vi "PH_Tektronix_7000.Configure Channel.vi"(0 "i ref in":refnum<vi>, 1 "Channel":u16(ring) items=["Channel 1", "Channel 2", "Channel 3", "Channel 4", "Math 1", "Math 2", "Math 3", "Math 4", "Reference 1", "Reference 2", "Reference 3", "Reference 4"], 2 "Channel Configuration":T1={"Enable Channel"=FALSE, "Bandwidth"=0, "Input Impedance"=0, "Vertical Coupling"=0, "Probe Attenuation"=1.0, "Range [V/div]"=1.0, "Position [div]"=10.0, "Bandwidth raw"=""} {"Vertical Coupling" items=["AC", "DC", "Ground"]; "Input Impedance" items=["1M", "50"]; "Bandwidth" items=["FULL", "500 MHz", "250 MHz", "150 MHz", "20 MHz"]}, 5 "error IO":errorcluster) -> (14 "i ref out":refnum<vi>, 19 "error out":errorcluster)   [LabVIEW 2014, in "PH_Tektronix_7000.lvlib"]
doc: "If the connection is established, the channel configuration is set and written to own attributes as well as the errors."
uses:
  PH_Tektronix_7000.lvlib
  PH_Tektronix_7000.Channel Config.ctl
  instr.lib/Tektronix7000Series/Tektronix 7000 Series - Driver np.lvlib
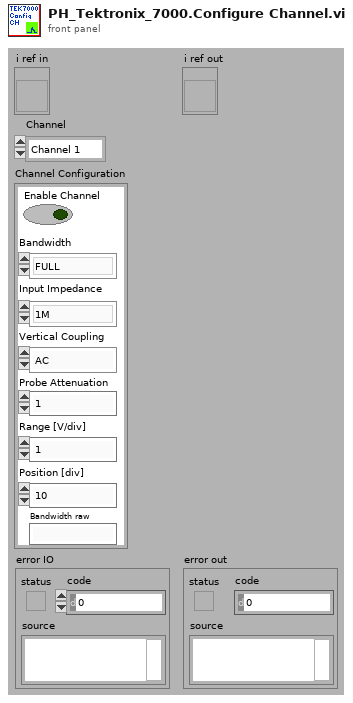
[diagram p1: front panel]
types:
  T1 = typedef "PH_Tektronix_7000.lvlib/PH_Tektronix_7000.Channel Config.ctl" = cluster{"Enable Channel":bool, "Bandwidth":u16, "Input Impedance":u16, "Vertical Coupling":u16, "Probe Attenuation":dbl, "Range [V/div]":dbl, "Position [div]":dbl, "Bandwidth raw":string}
  T2 = typedef "PH_Tektronix_7000.lvlib/PH_Tektronix_7000.i attribute.ctl" = cluster{"VISA Resource Name":refnum<visa-resource-name>, "IDN":cluster{"Instrument Driver":string, "Instrument Firmware":string, "Model":string, "Serial Number":string}, "Selftest":cluster{"Result":i32, "Message":string}, "Trigger Configuration":T3, "Acquisition Configuration":T4, "GUI Refs":T5, "State":T6, "Error Message":string, "Allow Prdc Loop?":bool, "Channel 1":T1, "Channel 2":T1, "Channel 3":T1, "Channel 4":T1, "Data CH 1":waveform(dbl), "Data CH 2":waveform(dbl), "Data CH 3":waveform(dbl), "Data CH 4":waveform(dbl), "Allow config?":bool, "Name Channel 1":string, "Name Channel 2":string, "Name Channel 3":string, "Name Channel 4":string, "Fetch Data before sending to PSDB?":bool, "Constructor passed?":bool, "Data taken at":timestamp, "Plot Colors":u32[], "Default VISA Resource":string}
  T3 = typedef "PH_Tektronix_7000.lvlib/PH_Tektronix_7000.Trigger Config.ctl" = cluster{"Source":u16, "Level [V]":dbl, "Slope":u16, "Coupling":u16, "Trigger Mode":u16}
  T4 = typedef "PH_Tektronix_7000.lvlib/PH_Tektronix_7000.Acquisition Config.ctl" = cluster{"Record Length":u32, "Timebase [s/div]":dbl, "Position [%]":dbl, "Acquisition Type":u16, "Average Waveforms":i32, "Envelope Waveforms":i32, "WfmDB Samples":i32, "Continuous?":bool, "Delay [s]":dbl, "Run?":bool}
  T5 = typedef "PH_Tektronix_7000.lvlib/PH_Tektronix_7000.GUI Refs.ctl" = cluster{"Graph":refnum<vi>, "State":refnum<vi>, "Delete":refnum<vi>, "VISA Resource":refnum<vi>, "Allow Configure":refnum<vi>, "Fetch Data":refnum<vi>, "Fetch before sending Data to PSDB":refnum<vi>, "Name Channel 1":refnum<vi>, "Name Channel 2":refnum<vi>, "Name Channel 3":refnum<vi>, "Name Channel 4":refnum<vi>, "Prdc Intervall [ms]":refnum<vi>, "Data taken":refnum<vi>, "Model":refnum<vi>, "Serial Number":refnum<vi>, "Firmware":refnum<vi>, "Driver":refnum<vi>, "Acquisition":refnum<vi>, "Trigger":refnum<vi>, "Cursor: D Time [s]":refnum<vi>, "Cursor: D Signal [V]":refnum<vi>, "Channel 1":refnum<vi>, "Channel 2":refnum<vi>, "Channel 3":refnum<vi>, "Channel 4":refnum<vi>}
  T6 = typedef "PH_StatusHandler.lvlib/PH_StatusHandler.Status.ctl" = i16
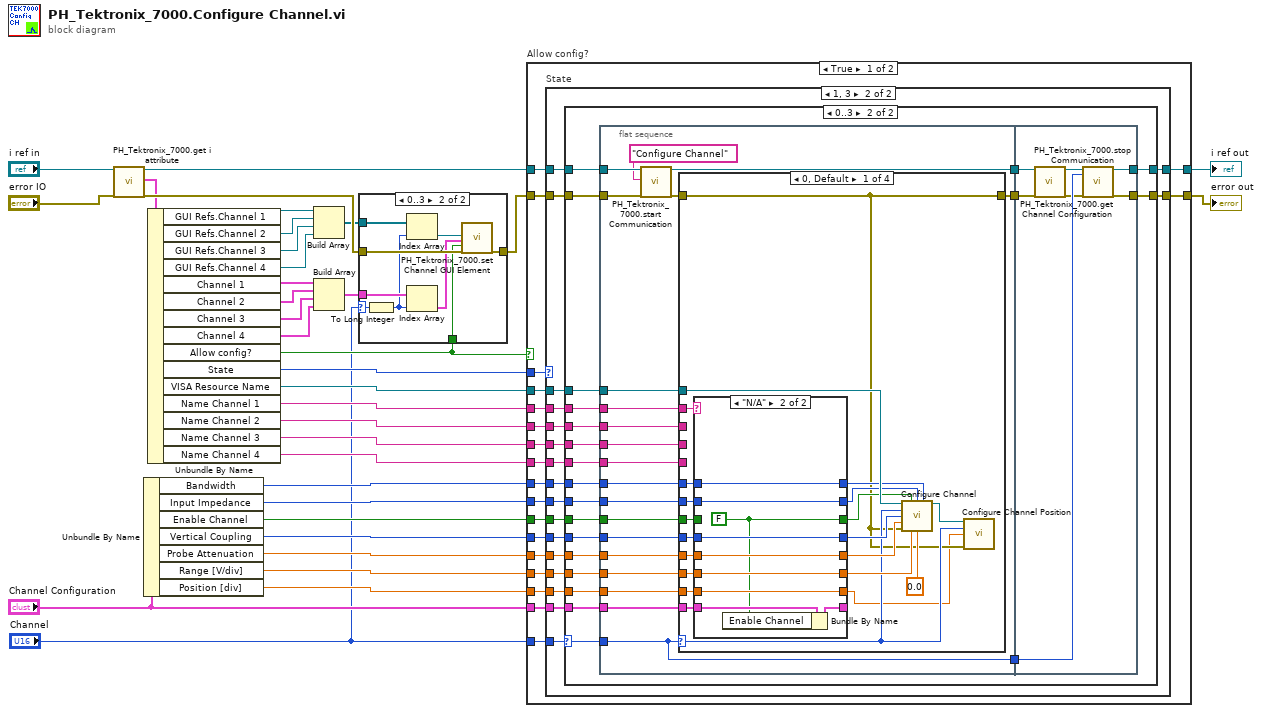
[diagram p0: block diagram]
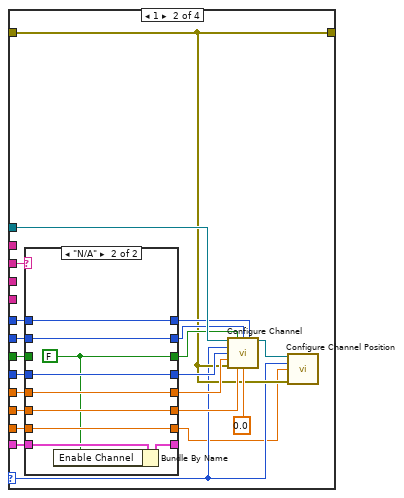
[diagram p6: hidden frame]
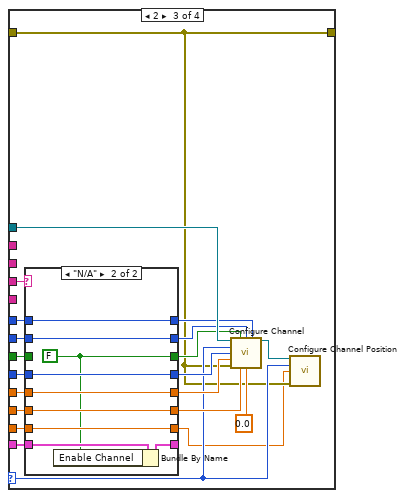
[diagram p8: hidden frame]
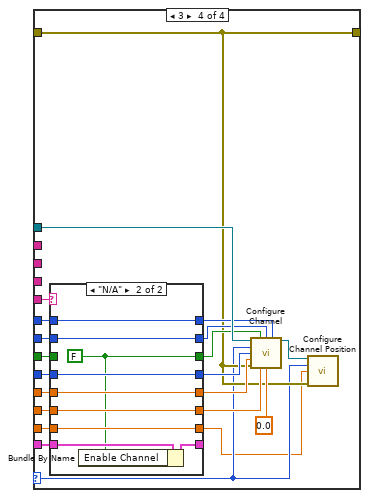
[diagram p10: hidden frame]
diagram:
  n1 = call "PH_Tektronix_7000.get i attribute.vi"("i ref in"="i ref in", "error in (no error)"="error IO") -> ("i ref out"=w30:refnum<vi>, "i attribute"=w32:T2, "error out"=w33:errorcluster)  [unwired: 15 in]
  n2 = Unbundle By Name("Channel Configuration") -> ("Bandwidth"=w27:u16, "Input Impedance"=w26:u16, "Enable Channel"=w25:bool, "Vertical Coupling"=w24:u16, "Probe Attenuation"=w23:dbl, "Range [V/div]"=w22:dbl, "Position [div]"=w21:dbl)
  n3 = Unbundle By Name(w32) -> ("GUI Refs.Channel 1"=w5:refnum<vi>, "GUI Refs.Channel 2"=w3:refnum<vi>, "GUI Refs.Channel 3"=w2:refnum<vi>, "GUI Refs.Channel 4"=w1:refnum<vi>, "Channel 1"=w7:T1, "Channel 2"=w10:T1, "Channel 3"=w9:T1, "Channel 4"=w8:T1, "Allow config?"=w12:bool, "State"=w13:T6, "VISA Resource Name"=w14:refnum<visa-resource-name>, "Name Channel 1"=w19:string, "Name Channel 2"=w18:string, "Name Channel 3"=w17:string, "Name Channel 4"=w16:string)
  n4 = Build Array(w5, w3, w2, w1) -> (w4:refnum<vi>[])
  n5 = Build Array(w7, w10, w9, w8) -> (w6:T1[])
  n6 = case shown="0..3" "Channel" {
    selector: "Channel" -> [_ w38]
    tunnel: w33 -> [w35 w44]
    tunnel: [w35 w43] -> w15
    tunnel: w12 -> [_ w42]
    tunnel: w4 -> [_ w41]
    tunnel: w6 -> [_ w40]
    frame Default {
    }
    frame 0..3 {
      n7 = To Long Integer(number=w38) -> (32bit integer=w36:i32)
      n8 = Index Array(array=w41, index=w36) -> (element=w37:refnum<vi>)
      n9 = Index Array(array=w40, index=w36) -> (element=w39:T1)
      n10 = call "PH_Tektronix_7000.set Channel GUI Element.vi"("GUI Ref Channel"=w37, "Channel Config"=w39, "enabled?"=w42, "error in"=w44) -> ("error out"=w43:errorcluster)  [unwired: 15 in]
    }
  }
  n11 = case "Allow config?" shown="True" w12 {
    tunnel: [w63 w287] -> w34
    tunnel: w15 -> [w62 w286]
    tunnel: w14 -> [w61 _]
    tunnel: w30 -> [w60 w287]
    tunnel: [w59 w286] -> w28
    tunnel: w27 -> [w58 _]
    tunnel: w26 -> [w57 _]
    tunnel: w25 -> [w56 _]
    tunnel: w24 -> [w55 _]
    tunnel: w23 -> [w54 _]
    tunnel: w22 -> [w53 _]
    tunnel: w21 -> [w52 _]
    tunnel: w13 -> [w45 _]
    tunnel: "Channel Configuration" -> [w51 _]
    tunnel: "Channel" -> [w46 _]
    tunnel: w19 -> [w50 _]
    tunnel: w18 -> [w49 _]
    tunnel: w17 -> [w48 _]
    tunnel: w16 -> [w47 _]
    frame True {
      n12 = case "State" shown="1, 3" w45 {
        tunnel: [w65 w66] -> w63
        tunnel: w62 -> [w64 w83]
        tunnel: w61 -> [_ w82]
        tunnel: w60 -> [w65 w67]
        tunnel: [w64 w81] -> w59
        tunnel: w58 -> [_ w80]
        tunnel: w57 -> [_ w79]
        tunnel: w56 -> [_ w78]
        tunnel: w55 -> [_ w77]
        tunnel: w54 -> [_ w76]
        tunnel: w53 -> [_ w75]
        tunnel: w52 -> [_ w74]
        tunnel: w51 -> [_ w73]
        tunnel: w50 -> [_ w72]
        tunnel: w49 -> [_ w71]
        tunnel: w48 -> [_ w70]
        tunnel: w47 -> [_ w69]
        tunnel: w46 -> [_ w68]
        frame Default {
        }
        frame 1, 3 {
          n13 = case shown="0..3" w68 {
            selector: w68 -> [_ w93]
            tunnel: w83 -> [w84 w91]
            tunnel: w82 -> [_ w106]
            tunnel: [w84 w87] -> w81
            tunnel: w80 -> [_ w105]
            tunnel: w79 -> [_ w104]
            tunnel: w78 -> [_ w103]
            tunnel: w77 -> [_ w102]
            tunnel: w76 -> [_ w101]
            tunnel: w75 -> [_ w100]
            tunnel: w74 -> [_ w99]
            tunnel: w73 -> [_ w98]
            tunnel: w72 -> [_ w97]
            tunnel: w71 -> [_ w96]
            tunnel: w70 -> [_ w95]
            tunnel: w69 -> [_ w94]
            tunnel: w67 -> [w85 w92]
            tunnel: [w85 w88] -> w66
            frame Default {
            }
            frame 0..3 {
              n14 = flat-sequence {
                tunnel: w106 -> [w126]
                tunnel: w105 -> [w125]
                tunnel: w104 -> [w124]
                tunnel: w103 -> [w123]
                tunnel: w102 -> [w122]
                tunnel: w101 -> [w121]
                tunnel: w100 -> [w120]
                tunnel: w99 -> [w119]
                tunnel: w98 -> [w118]
                tunnel: w97 -> [w117]
                tunnel: w96 -> [w116]
                tunnel: w95 -> [w115]
                tunnel: w94 -> [w114]
                tunnel: w93 -> [w107]
                tunnel: w92 -> [w113]
                tunnel: w91 -> [w112]
                tunnel: [w109] -> w90
                tunnel: [w108] -> w89
                tunnel: [w107] -> w86
                tunnel: [w284] -> w87
                tunnel: [w283] -> w88
                tunnel: w90 -> [w280]
                tunnel: w89 -> [w285]
                tunnel: w86 -> [w282]
                frame #0 {
                  n15 = call "PH_Tektronix_7000.start Communication.vi"("i ref in"=w113, "Action"="Configure Channel", "error in"=w112) -> ("i ref out"=w109:refnum<vi>, "error out"=w111:errorcluster)  [unwired: 15 in]
                  n16 = case "Channel Label" shown="0, Default" w107 {
                    selector: w107 -> [w130 w166 w205 w242]
                    tunnel: w111 -> [w128 w168 w204 w244]
                    tunnel: w126 -> [w147 w185 w223 w261]
                    tunnel: [w128 w168 w204 w244] -> w108
                    tunnel: w125 -> [w139 w183 w221 w260]
                    tunnel: w124 -> [w140 w182 w220 w259]
                    tunnel: w123 -> [w141 w181 w219 w258]
                    tunnel: w122 -> [w142 w180 w218 w257]
                    tunnel: w121 -> [w143 w179 w217 w256]
                    tunnel: w120 -> [w144 w178 w216 w255]
                    tunnel: w119 -> [w145 w177 w215 w254]
                    tunnel: w118 -> [w146 w176 w214 w253]
                    tunnel: w117 -> [w133 _ _ _]
                    tunnel: w116 -> [_ w184 _ _]
                    tunnel: w115 -> [_ _ w222 _]
                    tunnel: w114 -> [_ _ _ w252]
                    frame 0, Default {
                      n17 = case shown="\"N/A\"" w133 {
                        tunnel: w139 -> [w155 w164]
                        tunnel: [w155 w164] -> w135
                        tunnel: w140 -> [w154 w163]
                        tunnel: [w154 w163] -> w134
                        tunnel: w141 -> [w153 _]
                        tunnel: [w153 w157] -> w136
                        tunnel: w142 -> [w152 w162]
                        tunnel: [w152 w162] -> w132
                        tunnel: w143 -> [w151 w161]
                        tunnel: [w151 w161] -> w137
                        tunnel: w144 -> [w150 w160]
                        tunnel: [w150 w160] -> w138
                        tunnel: w145 -> [w149 w159]
                        tunnel: [w149 w159] -> w127
                        tunnel: w146 -> [w148 w158]
                        tunnel: [w148 w156] -> _
                        frame Default {
                        }
                        frame "N/A" {
                          w157 = FALSE
                          n18 = Bundle By Name(cluster=w158, "Enable Channel"=w157) -> (w156:T1)
                        }
                      }
                      n19 = call "Configure Channel.vi"("VISA resource name"=w147, "Enable Channel (T: Enable)"=w136, "Input Impedance (0: 1M ohm)"=w134, "Bandwidth (0: FULL)"=w135, "Channel (0: Channel 1)"=w130, "Vertical Coupling (1: DC)"=w132, "Probe Attenuation (1.0)"=w137, "error in (no error)"=w128, "Vertical Range (10.0 V)"=w138, "Vertical Offset (0.0 V)"=0.0) -> ("VISA resource name out"=w129:refnum<visa-resource-name>)  [unwired: 4 in, 1 out]
                      n20 = call "Configure Channel Position.vi"("VISA resource name"=w129, "Channel (0: Channel 1)"=w130, "Vertical Position (0.0 div)"=w127, "error in (no error)"=w128) -> ()  [unwired: 10 in, 2 out]
                    }
                    frame 1 {
                      n21 = case shown="\"N/A\"" w184 {
                        tunnel: w183 -> [w193 w202]
                        tunnel: [w193 w202] -> w175
                        tunnel: w182 -> [w192 w201]
                        tunnel: [w192 w201] -> w174
                        tunnel: w181 -> [w191 _]
                        tunnel: [w191 w195] -> w173
                        tunnel: w180 -> [w190 w200]
                        tunnel: [w190 w200] -> w172
                        tunnel: w179 -> [w189 w199]
                        tunnel: [w189 w199] -> w171
                        tunnel: w178 -> [w188 w198]
                        tunnel: [w188 w198] -> w170
                        tunnel: w177 -> [w187 w197]
                        tunnel: [w187 w197] -> w165
                        tunnel: w176 -> [w186 w196]
                        tunnel: [w186 w194] -> _
                        frame Default {
                        }
                        frame "N/A" {
                          w195 = FALSE
                          n22 = Bundle By Name(cluster=w196, "Enable Channel"=w195) -> (w194:T1)
                        }
                      }
                      n23 = call "Configure Channel.vi"("VISA resource name"=w185, "Enable Channel (T: Enable)"=w173, "Input Impedance (0: 1M ohm)"=w174, "Bandwidth (0: FULL)"=w175, "Channel (0: Channel 1)"=w166, "Vertical Coupling (1: DC)"=w172, "Probe Attenuation (1.0)"=w171, "error in (no error)"=w168, "Vertical Range (10.0 V)"=w170, "Vertical Offset (0.0 V)"=0.0) -> ("VISA resource name out"=w167:refnum<visa-resource-name>)  [unwired: 4 in, 1 out]
                      n24 = call "Configure Channel Position.vi"("VISA resource name"=w167, "Channel (0: Channel 1)"=w166, "Vertical Position (0.0 div)"=w165, "error in (no error)"=w168) -> ()  [unwired: 10 in, 2 out]
                    }
                    frame 2 {
                      n25 = case shown="\"N/A\"" w222 {
                        tunnel: w221 -> [w231 w240]
                        tunnel: [w231 w240] -> w213
                        tunnel: w220 -> [w230 w239]
                        tunnel: [w230 w239] -> w212
                        tunnel: w219 -> [w229 _]
                        tunnel: [w229 w233] -> w211
                        tunnel: w218 -> [w228 w238]
                        tunnel: [w228 w238] -> w210
                        tunnel: w217 -> [w227 w237]
                        tunnel: [w227 w237] -> w209
                        tunnel: w216 -> [w226 w236]
                        tunnel: [w226 w236] -> w208
                        tunnel: w215 -> [w225 w235]
                        tunnel: [w225 w235] -> w203
                        tunnel: w214 -> [w224 w234]
                        tunnel: [w224 w232] -> _
                        frame Default {
                        }
                        frame "N/A" {
                          w233 = FALSE
                          n26 = Bundle By Name(cluster=w234, "Enable Channel"=w233) -> (w232:T1)
                        }
                      }
                      n27 = call "Configure Channel.vi"("VISA resource name"=w223, "Enable Channel (T: Enable)"=w211, "Input Impedance (0: 1M ohm)"=w212, "Bandwidth (0: FULL)"=w213, "Channel (0: Channel 1)"=w205, "Vertical Coupling (1: DC)"=w210, "Probe Attenuation (1.0)"=w209, "error in (no error)"=w204, "Vertical Range (10.0 V)"=w208, "Vertical Offset (0.0 V)"=0.0) -> ("VISA resource name out"=w206:refnum<visa-resource-name>)  [unwired: 4 in, 1 out]
                      n28 = call "Configure Channel Position.vi"("VISA resource name"=w206, "Channel (0: Channel 1)"=w205, "Vertical Position (0.0 div)"=w203, "error in (no error)"=w204) -> ()  [unwired: 10 in, 2 out]
                    }
                    frame 3 {
                      n29 = case shown="\"N/A\"" w252 {
                        tunnel: w260 -> [w269 w278]
                        tunnel: [w269 w278] -> w251
                        tunnel: w259 -> [w268 w277]
                        tunnel: [w268 w277] -> w250
                        tunnel: w258 -> [w267 _]
                        tunnel: [w267 w271] -> w249
                        tunnel: w257 -> [w266 w276]
                        tunnel: [w266 w276] -> w248
                        tunnel: w256 -> [w265 w275]
                        tunnel: [w265 w275] -> w247
                        tunnel: w255 -> [w264 w274]
                        tunnel: [w264 w274] -> w246
                        tunnel: w254 -> [w263 w273]
                        tunnel: [w263 w273] -> w241
                        tunnel: w253 -> [w262 w272]
                        tunnel: [w262 w270] -> _
                        frame Default {
                        }
                        frame "N/A" {
                          w271 = FALSE
                          n30 = Bundle By Name(cluster=w272, "Enable Channel"=w271) -> (w270:T1)
                        }
                      }
                      n31 = call "Configure Channel.vi"("VISA resource name"=w261, "Enable Channel (T: Enable)"=w249, "Input Impedance (0: 1M ohm)"=w250, "Bandwidth (0: FULL)"=w251, "Channel (0: Channel 1)"=w242, "Vertical Coupling (1: DC)"=w248, "Probe Attenuation (1.0)"=w247, "error in (no error)"=w244, "Vertical Range (10.0 V)"=w246, "Vertical Offset (0.0 V)"=0.0) -> ("VISA resource name out"=w243:refnum<visa-resource-name>)  [unwired: 4 in, 1 out]
                      n32 = call "Configure Channel Position.vi"("VISA resource name"=w243, "Channel (0: Channel 1)"=w242, "Vertical Position (0.0 div)"=w241, "error in (no error)"=w244) -> ()  [unwired: 10 in, 2 out]
                    }
                  }
                }
                frame #1 {
                  n33 = call "PH_Tektronix_7000.stop Communication.vi"("i ref in"=w280, "error in"=w285) -> ("i ref out"=w279:refnum<vi>, "error out"=w281:errorcluster)  [unwired: 16 in]
                  n34 = call "PH_Tektronix_7000.get Channel Configuration.vi"("i ref in"=w279, "Channel"=w282, "error IO"=w281) -> ("i ref out"=w283:refnum<vi>, "error out"=w284:errorcluster)  [unwired: 15 in]
                }
              }
            }
          }
        }
      }
    }
    frame False {
    }
  }
  "i ref out" <- w34
  "error out" <- w28
